vi "Check Valid UI Selection.vi"(8 "error in (no error)":errorcluster, 11 "Operator UI in":refnum<class "Measurement Setup UI.lvclass">) -> (0 "error out":errorcluster, 3 "Operator UI out":refnum<class "Measurement Setup UI.lvclass">)   [LabVIEW 2016, in "Measurement Setup Controller.lvlib" / "Measurement Setup UI.lvclass"]
uses:
  Measurement Setup UI.lvclass
  \\Mac\Home/Documents/MAL-Framework/user.lib/Common Components/Msmt UI/Measurement UI.lvclass
  Measurement Setup UI.lvclass/Measurement Setup UI.ctl
  MAL-Framework/user.lib/Common Components/Msmt UI/Measurement UI.lvclass/Measurement UI.ctl
  Read Save.vi
  MAL-Framework/user.lib/Common Components/Msmt UI/Accessors/Read Run.vi
  MAL-Framework/user.lib/Common Components/Msmt UI/Measurement UI.lvclass
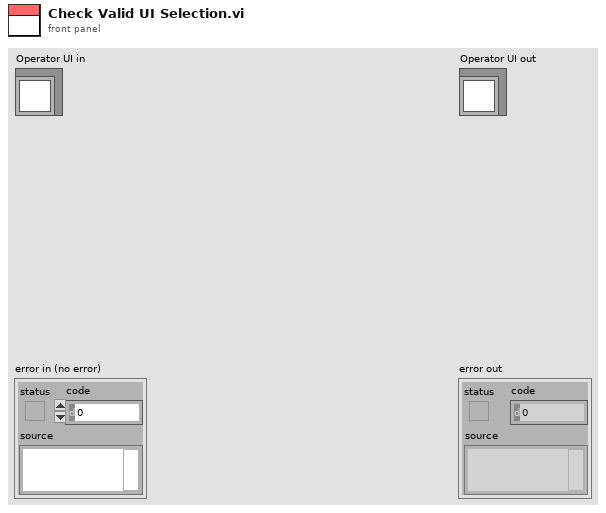
[diagram p1: front panel]
types:
  T1 = enum8{"Enabled", "Disabled", "Disabled and Grayed Out"}
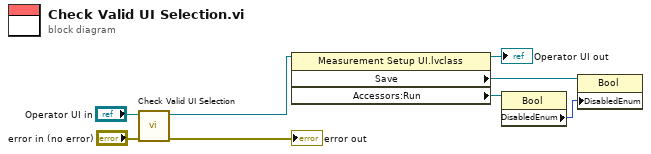
[diagram p0: block diagram]
diagram:
  n1 = call-parent "Check Valid UI Selection.vi"("error in (no error)"="error in (no error)", "Operator UI in"="Operator UI in") -> ("error out"=→"error out":errorcluster, "Operator UI out"=w7:refnum<class "Measurement Setup UI.lvclass">)  [unwired: 8 in]
  n2 = property class="Measurement Setup UI.lvclass"(reference=w7) -> (reference out=→"Operator UI out":refnum<class "Measurement Setup UI.lvclass">, "Save"=w3:refnum<vi>, "Accessors:Run"=w1:refnum<vi>)  [unwired: 1 in, 1 out]
  n3 = property class="Bool"(reference=w1) -> ("DisabledEnum"=w2:T1)  [unwired: 1 in, 2 out]
  n4 = property class="Bool"(reference=w3, "DisabledEnum"=w2) -> ()  [unwired: 1 in, 2 out]
